vi "Init ECAT Reconfig VI.vi"(8 "error in (no error)":errorcluster, 11 "ECAT Modules":T2[](array[typedef])) -> (0 "error out":errorcluster, 3 "ECAT Reconfig out":T1)   [LabVIEW 2016, in "Scan Engine Custom Device.lvlib"]
uses:
  Scan Engine Custom Device.lvlib
  Type Defs/ECAT Reconfig State.ctl
  Type Defs/ECAT Reconfig Status.ctl
  Type Defs/ECAT Reconfig Data.ctl
  Read-Write/Reconfig ECAT Modules.vi
  Modules.lvlibp/RSI Module/RSI Module.lvclass
  Type Defs/ECAT Module Reconfig.ctl
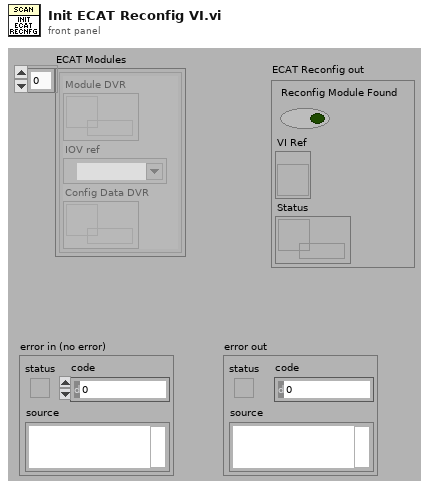
[diagram p1: front panel]
types:
  T1 = typedef "Scan Engine Custom Device.lvlib/ECAT Reconfig Data.ctl" = cluster{"Reconfig Module Found":bool, "VI Ref":refnum<vi>, "Status":refnum<queue>}
  T2 = typedef "Scan Engine Custom Device.lvlib/ECAT Module Reconfig.ctl" = cluster{"Module DVR":refnum<data-value>, "IOV ref":refnum<k21>, "Config Data DVR":refnum<data-value>}
  T3 = typedef "Scan Engine Custom Device.lvlib/ECAT Reconfig State.ctl" = enum16{"Not running", "Waiting to Start", "Started", "Running"}
  T4 = typedef "Scan Engine Custom Device.lvlib/ECAT Reconfig Status.ctl" = cluster{"State":T3, "error":errorcluster}
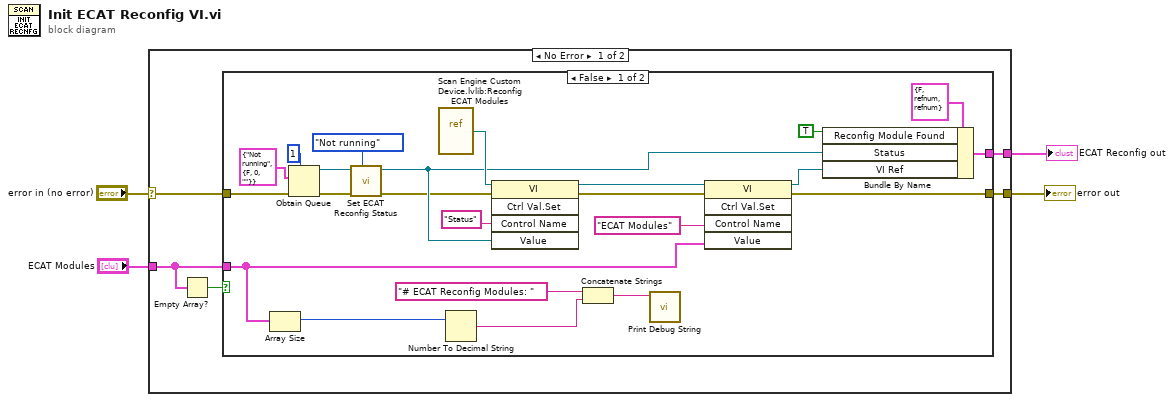
[diagram p0: block diagram]
diagram:
  n1 = case shown="No Error" "error in (no error)" {
    selector: "error in (no error)" -> [w9 w34]
    tunnel: "ECAT Modules" -> [w6 _]
    tunnel: [w8 w34] -> w4
    tunnel: [w5 _] -> w1
    frame No Error {
      n2 = Empty Array?(array=w6) -> (empty?=w7:bool)
      n3 = case shown="False" w7 {
        tunnel: w6 -> [w22 _]
        tunnel: w9 -> [w26 w33]
        tunnel: [w25 w33] -> w8
        tunnel: [w17 _] -> w5
        frame False {
          n4 = Array Size(array=w22) -> (size(s)=w21:i32)
          n5 = Obtain Queue(max queue size (-1, unlimited)=1, element data type=T4 {"State"=enum."Not running", "error"={"status"=FALSE, "code"=0, "source"=""}} ("ECAT Reconfig Status"), error in (no error)=w26) -> (queue out=w10:refnum<queue>, error out=w15:errorcluster)  [unwired: 2 in, 1 out]
          n6 = call "Set ECAT Reconfig Status.vi"("State"=ECAT_Reconfig_State."Not running", "error in (no error)"=w15, "Status in"=w10) -> ("error out"=w12:errorcluster, "Status out"=w14:refnum<queue>)  [unwired: 7 in]
          n7 = vi-ref "Scan Engine Custom Device.lvlib:Reconfig ECAT Modules.vi"() -> (w27:refnum<vi>)
          n8 = Number To Decimal String(number=w21) -> (decimal integer string=w20:string)  [unwired: 1 in]
          n9 = invoke class="VI" method="Ctrl Val.Set"(reference=w27, error in=w12, "Control Name"="Status", "Value"=w14) -> (reference out=w28:refnum<vi>, error out=w29:errorcluster)  [unwired: 1 in, 3 out]
          n10 = Concatenate Strings("# ECAT Reconfig Modules: ", w20) -> (w23:string)
          n11 = call "Print Debug String.vi"("String to write"=w23) -> ()  [unwired: 9 in, 1 out]
          n12 = invoke class="VI" method="Ctrl Val.Set"(reference=w28, error in=w29, "Control Name"="ECAT Modules", "Value"=w22) -> (reference out=w16:refnum<vi>, error out=w25:errorcluster)  [unwired: 1 in, 3 out]
          n13 = Bundle By Name(cluster=T1 {"Reconfig Module Found"=FALSE, "VI Ref"=refnum, "Status"=refnum} ("ECAT Reconfig out"), "Reconfig Module Found"=TRUE, "Status"=w14, "VI Ref"=w16) -> (w17:T1)
        }
        frame True {
        }
      }
    }
    frame Error {
    }
  }
  "error out" <- w4
  "ECAT Reconfig out" <- w1
